vi "getComputerName.vi"() -> (1 "full name":string, 2 "name":string, 3 "IP":string)   [LabVIEW 2017]
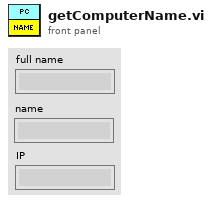
[diagram p1: front panel]
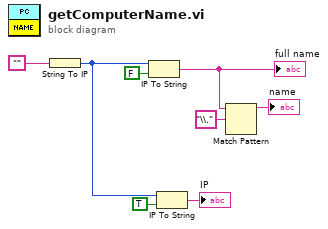
[diagram p0: block diagram]
diagram:
  n1 = String To IP(1:"") -> (0:w6:u32)
  n2 = IP To String(1:FALSE ("dot notation? (F)"), 2:w6) -> (0:w4:string)
  "full name" <- w4
  n3 = IP To String(1:TRUE ("dot notation? (F)"), 2:w6) -> (0:→"IP":string)
  n4 = Match Pattern(string=w4, regular expression="\\.") -> (before substring=→"name":string)  [unwired: 1 in, 3 out]
